vi "WriteRebootLogLine.vi"(8 "error in":errorcluster, 9 "reboot log text":string, 10 "operation":T1, 11 "log path":path) -> (0 "error out":errorcluster, 3 "log path out":path)   [LabVIEW 2017, in "Controller.lvlib"]
uses:
  <vilib>/addons/InsightCM/Devices/Shared/Common/Controller/Controller.lvlib
  <vilib>/addons/InsightCM/Devices/Shared/Common/Controller/controls/operations.ctl
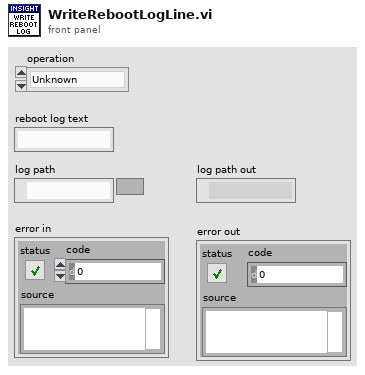
[diagram p1: front panel]
types:
  T1 = typedef "Controller.lvlib/operations.ctl" = enum16{"Unknown", "Startup", "Expected Shutdown"}
  T2 = enum16{"open", "replace", "create", "open or create", "replace or create", "replace or create with confirmation"}
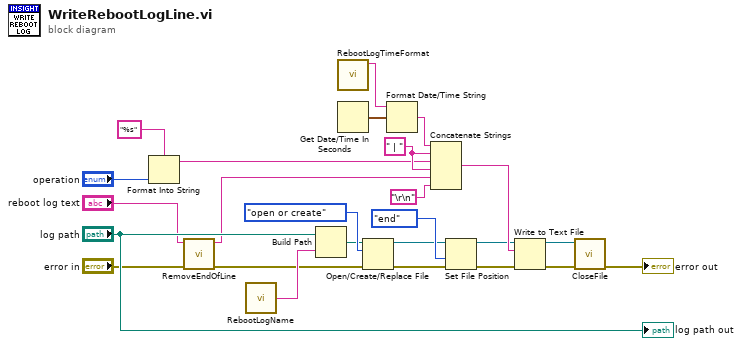
[diagram p0: block diagram]
diagram:
  w12 = " | " ("string")
  n1 = Format Into String(format string="%s", "operation") -> (resulting string=w9:string)  [unwired: 2 in, 1 out]
  n2 = call <vilib>:"RemoveEndOfLine.vi"("error in"="error in", "reboot log text"="reboot log text") -> ("error out"=w6:errorcluster, "reboot log text out"=w4:string)  [unwired: 8 in]
  n3 = call <vilib>:"RebootLogName.vi"() -> ("reboot log name"=w14:string)  [unwired: 5 in]
  n4 = Build Path(base path="log path", name or relative path=w14) -> (appended path=w15:path)
  n5 = call <vilib>:"RebootLogTimeFormat.vi"() -> ("time format"=w8:string)  [unwired: 11 in]
  n6 = Get Date/Time In Seconds() -> (seconds since 1Jan1904=w25:timestamp)
  n7 = Open/Create/Replace File(file path (use dialog)=w15, error in=w6, operation (0:open)=T2."open or create") -> (refnum out=w18:refnum<file>, error out=w20:errorcluster)  [unwired: 3 in, 1 out]
  n8 = Format Date/Time String(time format string (%c)=w8, seconds (now)=w25) -> (date/time string=w24:string)  [unwired: 1 in]
  n9 = Concatenate Strings(w24, w12, w9, w12, w4, "\r\n") -> (w23:string)
  n10 = Set File Position(refnum=w18, from (0:start)=enum16{"start", "end", "current"}."end", error in=w20) -> (refnum out=w21:refnum<file>, error out=w22:errorcluster)  [unwired: 1 in]
  n11 = Write to Text File(file (use dialog)=w21, text=w23, error in=w22) -> (refnum out=w3:refnum<file>, error out=w2:errorcluster)  [unwired: 1 in, 1 out]
  n12 = call <vilib>:"CloseFile.vi"("error in (no error)"=w2, "file reference"=w3) -> ("error out"=→"error out":errorcluster)  [unwired: 9 in]
  "log path out" <- "log path"
